vi "Distribute.vi"(8 "error in (no error)":errorcluster, 10 "Bounds":T1, 11 "Container in":refnum<class "Viewport.lvclass">) -> (0 "error out":errorcluster, 2 "Bounds":T1[](array[typedef]), 3 "Container out":refnum<class "Viewport.lvclass">, 5 "Visible bounds":T1[](array[typedef]), 7 "Visible indices":i32[](array[numeric]))   [LabVIEW 2013, in "Viewport.lvclass"]
doc: "Copyright 2018, Wiebe Walstra, wiebe@carya.nl."
uses:
  Viewport.lvclass
  <vilib>/Utility/miscctls.llb/LVRectTypeDef.ctl
  IContainer.lvclass
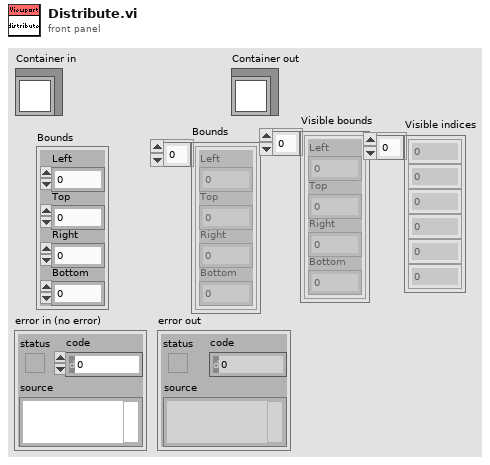
[diagram p1: front panel]
types:
  T1 = typedef "LVRectTypeDef.ctl" = cluster{"Left":i16, "Top":i16, "Right":i16, "Bottom":i16}
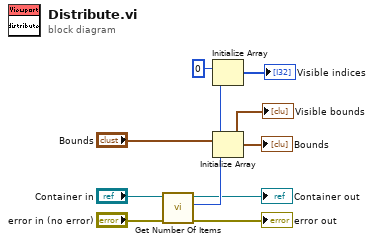
[diagram p0: block diagram]
diagram:
  n1 = call "Get Number Of Items.vi"("error in (no error)"="error in (no error)", "IContainer in"="Container in") -> ("error out"=→"error out":errorcluster, "Items"=w5:i32, "IContainer out"=→"Container out":refnum<class "Viewport.lvclass">)  [unwired: 7 in]
  n2 = Initialize Array(0, w5) -> (→"Visible indices":i32[])
  n3 = Initialize Array("Bounds", w5) -> (→"Bounds" →"Visible bounds":T1[])
